vi "Get Pulse.vi"(7 "Channel (1: Chan A)":i32(ring)=1 items=["Channel A"=1, "Channel B"=2, "Channel C"=3, "Channel D"=4, "Channel E"=5, "Channel F"=6, "Channel G"=7, "Channel H"=8], 8 "error in (no error)":errorcluster, 11 "VISA resource name":refnum<visa-resource-name>) -> (0 "error out":errorcluster, 1 "Width":dbl=nan format="%.6p", 2 "Delay":dbl=nan format="%.6p", 3 "VISA resource name out":refnum<visa-resource-name>, 5 "Wait #":i32=-1)   [LabVIEW 2012, in "Berkeley Nucleonics 500 Series.lvlib"]
doc: "This VI is used to read the pulse configuration of the selected channel."
uses:
  Berkeley Nucleonics 500 Series.lvlib
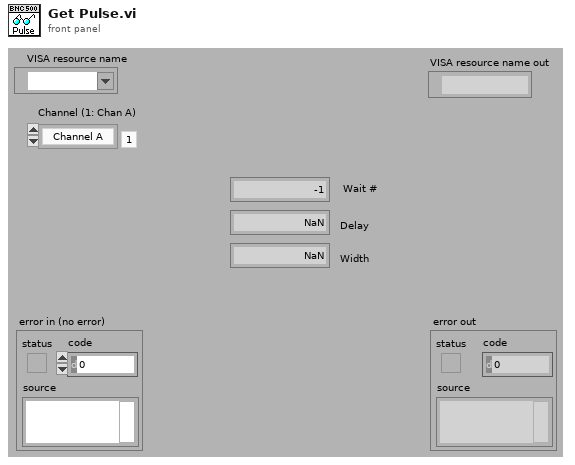
[diagram p1: front panel]
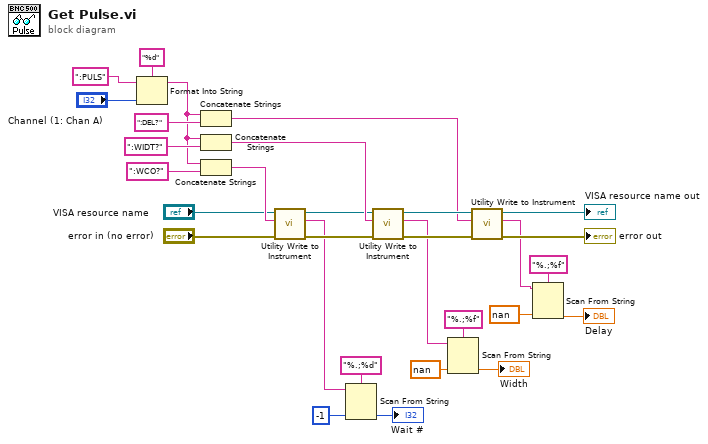
[diagram p0: block diagram]
diagram:
  n1 = Format Into String(format string="%d", initial string=":PULS", "Channel (1: Chan A)") -> (resulting string=w6:string)  [unwired: 1 in, 1 out]
  n2 = Concatenate Strings(w6, ":DEL?") -> (w16:string)
  n3 = Concatenate Strings(w6, ":WIDT?") -> (w17:string)
  n4 = Concatenate Strings(w6, ":WCO?") -> (w7:string)
  n5 = call "Utility Write to Instrument.vi"("error in (no error)"="error in (no error)", "Write Buffer"=w7, "VISA resource name"="VISA resource name") -> ("error out"=w12:errorcluster, "Read Buffer"=w8:string, "VISA resource name out"=w13:refnum<visa-resource-name>)  [unwired: 6 out]
  n6 = Scan From String(format string="%.;%d", input string=w8, default 1=-1 ("default value 1")) -> (output 1=→"Wait #":i32)  [unwired: 2 in, 3 out]
  n7 = call "Utility Write to Instrument.vi"("error in (no error)"=w12, "Write Buffer"=w17, "VISA resource name"=w13) -> ("error out"=w22:errorcluster, "Read Buffer"=w21:string, "VISA resource name out"=w23:refnum<visa-resource-name>)  [unwired: 6 out]
  n8 = Scan From String(format string="%.;%f", input string=w21, default 1=nan ("default value 1")) -> (output 1=→"Width":dbl)  [unwired: 2 in, 3 out]
  n9 = call "Utility Write to Instrument.vi"("error in (no error)"=w22, "Write Buffer"=w16, "VISA resource name"=w23) -> ("error out"=→"error out":errorcluster, "Read Buffer"=w18:string, "VISA resource name out"=→"VISA resource name out":refnum<visa-resource-name>)  [unwired: 6 out]
  n10 = Scan From String(format string="%.;%f", input string=w18, default 1=nan ("default value 1")) -> (output 1=→"Delay":dbl)  [unwired: 2 in, 3 out]
